vi "GetAlpha.vi"(8 "error in (no error)":errorcluster, 11 "ColorRGBA in":refnum<class "ColorRGBA.lvclass">) -> (0 "error out":errorcluster, 2 "Alpha":u8, 3 "ColorRGBA out":refnum<class "ColorRGBA.lvclass">)   [LabVIEW 2021, in "Picture2D.lvlib" / "ColorRGBA.lvclass"]
uses:
  ColorRGBA.lvclass
  ColorRGBA.lvclass/ColorRGBA.ctl
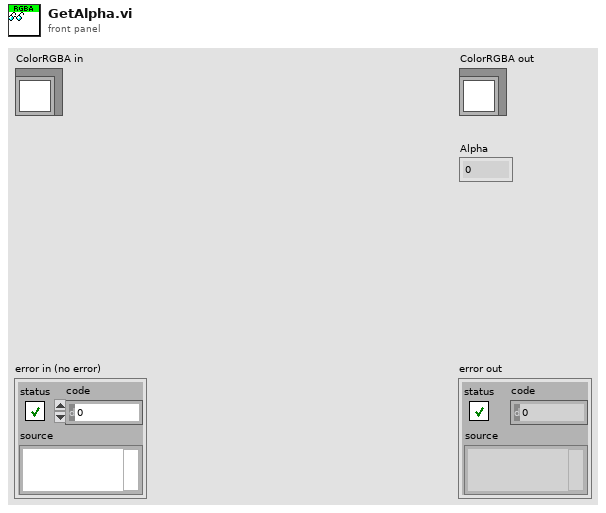
[diagram p1: front panel]
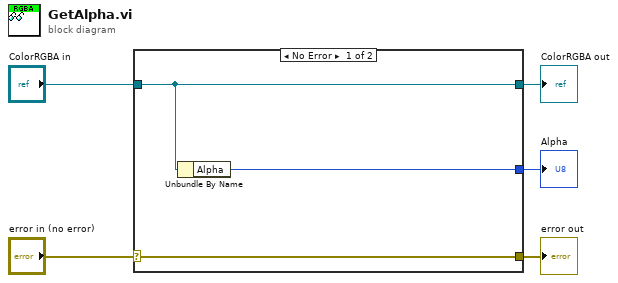
[diagram p0: block diagram]
diagram:
  n1 = case shown="No Error" "error in (no error)" {
    selector: "error in (no error)" -> [w8 w9]
    tunnel: [w8 w9] -> w4
    tunnel: [w7 w10] -> w2
    tunnel: "ColorRGBA in" -> [w7 w10]
    tunnel: [w6 _] -> w1
    frame No Error {
      n2 = Unbundle By Name(w7) -> ("Alpha"=w6:u8)
    }
    frame Error {
    }
  }
  "error out" <- w4
  "ColorRGBA out" <- w2
  "Alpha" <- w1
